vi "Reset ROI.vi"(8 "error in (no error)":errorcluster, 11 "TG Base Graph in":refnum<class "Base Graph.lvclass">) -> (0 "error out":errorcluster, 3 "TG Base Graph out":refnum<class "Base Graph.lvclass">)   [LabVIEW 2023, in "Base Graph.lvclass"]
uses:
  Base Graph.lvclass
  Base Graph.lvclass/Base Graph.ctl
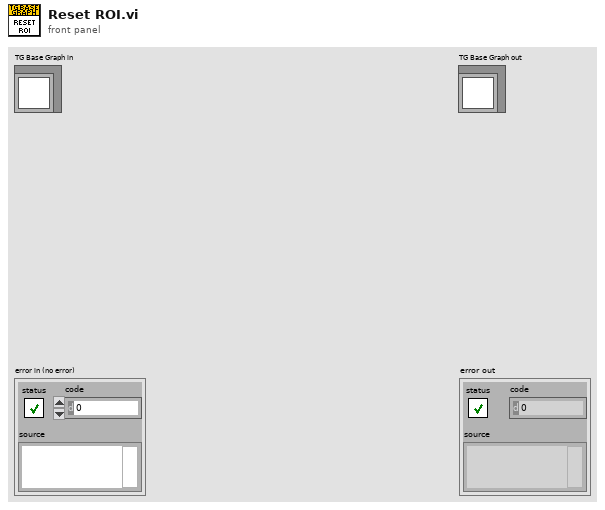
[diagram p1: front panel]
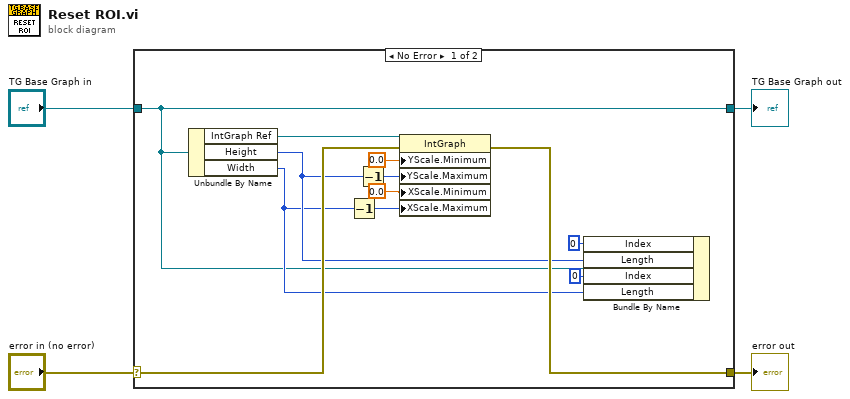
[diagram p0: block diagram]
diagram:
  n1 = case shown="No Error" "error in (no error)" {
    selector: "error in (no error)" -> [w15 w18]
    tunnel: [w12 w18] -> w3
    tunnel: [w7 w17] -> w1
    tunnel: "TG Base Graph in" -> [w7 w17]
    frame No Error {
      n2 = Unbundle By Name(w7) -> ("IntGraph Ref"=w16:refnum<vi>, "Height"=w9:u32, "Width"=w8:u32)
      n3 = Decrement(x=w8) -> (x-1=w5:u32)
      n4 = Decrement(x=w9) -> (x-1=w6:u32)
      n5 = property class="IntGraph"(reference=w16, error in=w15, "YScale.Minimum"=0.0 ("Y Scale.Range:Minimum"), "YScale.Maximum"=w6, "XScale.Minimum"=0.0 ("X Scale.Range:Minimum"), "XScale.Maximum"=w5) -> (error out=w12:errorcluster)  [unwired: 1 out]
      n6 = Bundle By Name(cluster=w7, "Index"=u32 0 ("ROI XY.ROI X.Index"), "Length"=w9, "Index"=u32 0 ("ROI XY.ROI Y.Index"), "Length"=w8) -> ()  [unwired: 1 out]
    }
    frame Error {
    }
  }
  "error out" <- w3
  "TG Base Graph out" <- w1
